vi "AquaLogic_Test_Stand.vi"() -> ()   [LabVIEW 2011]
panel:
  in  "Save Interval [s]":dbl=30.0 min=0.0
  in  "Save Enable":bool
  in  "STOP PROGRAM":bool
  in  "MAIN TAB":T1(tab)
  in  "?":T2={"ON-DEMAND Display"=[{"CMD_Display"="User Parameter : 20 Conductivity Thresholds", "Parameter Table"=[[">= Water Presence", ">= Low Salt", "<= Out of Salt [OFF]"], ["08.000", "10.000", "12.000"]], "SET"=FALSE, "GET"=FALSE}, {"CMD_Display"="User Parameter : 22 PCB Temp Threshold", "Parameter Table"=[[">= Max PCB Temp (°F)", "", ""], ["200.00", "", ""]], "SET"=FALSE, "GET"=FALSE}, {"CMD_Display"="User Parameter : 24 DayTank Setpoints", "Parameter Table"=[["<= Min / Empty Tank", ">= Fill Setpoint", ">= Tank Overfill"], ["00.500", "00.750", "01.250"]], "SET"=FALSE, "GET"=FALSE}, {"CMD_Display"="User Parameter : 25 Voltage Thresholds", "Parameter Table"=[["<= Min / Failure", ">= Low Salt", ">= Max / Failure"], ["00.000", "15.000", "20.000"]], "SET"=FALSE, "GET"=FALSE}, {"CMD_Display"="User Parameter : 26 Current Setpoint Limits", "Parameter Table"=[["Minimum Current (amps)", "Maximum Current (amps)", ""], ["00.000", "15.000", ""]], "SET"=FALSE, "GET"=FALSE}, {"CMD_Display"="User Parameter : 27 CURRCELL PWM Ramp", "Parameter Table"=[["Ramp Up Rate", "Ramp Down Rate", ""], ["00.250", "15.000", ""]], "SET"=FALSE, "GET"=FALSE}, {"CMD_Display"="User Parameter : 28 OUTPUT PWM Ramp", "Parameter Table"=[["Ramp Up Rate", "Ramp Down Rate", ""], ["00.500", "01.000", ""]], "SET"=FALSE, "GET"=FALSE}, {"CMD_Display"="User Parameter : 29 Cell Current SP / Status", "Parameter Table"=[["CURRCELL SP (amps)", "", ""], ["00.000", "", ""]], "SET"=FALSE, "GET"=FALSE}, {"CMD_Display"="User Parameter : 30 PWM Output 1 Setpoint", "Parameter Table"=[["Duty Cycle SP (%)", "", ""], ["0.00", "", ""]], "SET"=FALSE, "GET"=FALSE}, {"CMD_Display"="User Parameter : 31 PWM Output 2 Setpoint", "Parameter Table"=[["Duty Cycle SP (%)", "", ""], ["000.00", "", ""]], "SET"=FALSE, "GET"=FALSE}, {"CMD_Display"="User Parameter : 32 PWM Output 3 Setpoint", "Parameter Table"=[["Duty Cycle SP (%)", "", ""], ["000.00", "", ""]], "SET"=FALSE, "GET"=FALSE}], "CONTINUOUS Display"=[{"CMD_Display"="DU:33  Cell Status", "Param Output"=[["CELLDRIVE Duty (%)", "VOLTSCELL (volts)", "CURRCELL (amps)"], ["000.00", "00.000", "00.015"]]}, {"CMD_Display"="DU:34  PWM1 Status", "Param Output"=[["Duty Cycle (%)", "EMFOUT (volts)", "OVRCOUT (amps)"], ["000.00", "00.765", "00.000"]]}, {"CMD_Display"="DU:41  Temperature Measurements", "Param Output"=[["PCB Temperature (°F)", "Conductivity Temp (°F)", ""], ["069.91", "Conductivity Temp (°F)", ""]]}], "ERROR List"=[], "STATUS List"=[], "DIGITAL List"=[]}
  in  "Display B":T2={"ON-DEMAND Display"=[{"CMD_Display"="User Parameter : 20 Conductivity Thresholds", "Parameter Table"=[[">= Water Presence", ">= Low Salt", "<= Out of Salt [OFF]"], ["08.000", "10.000", "12.000"]], "SET"=FALSE, "GET"=FALSE}, {"CMD_Display"="User Parameter : 22 PCB Temp Threshold", "Parameter Table"=[[">= Max PCB Temp (°F)", "", ""], ["200.00", "", ""]], "SET"=FALSE, "GET"=FALSE}, {"CMD_Display"="User Parameter : 24 DayTank Setpoints", "Parameter Table"=[["<= Min / Empty Tank", ">= Fill Setpoint", ">= Tank Overfill"], ["00.500", "00.750", "01.250"]], "SET"=FALSE, "GET"=FALSE}, {"CMD_Display"="User Parameter : 25 Voltage Thresholds", "Parameter Table"=[["<= Min / Failure", ">= Low Salt", ">= Max / Failure"], ["00.000", "15.000", "20.000"]], "SET"=FALSE, "GET"=FALSE}, {"CMD_Display"="User Parameter : 26 Current Setpoint Limits", "Parameter Table"=[["Minimum Current (amps)", "Maximum Current (amps)", ""], ["00.000", "15.000", ""]], "SET"=FALSE, "GET"=FALSE}, {"CMD_Display"="User Parameter : 27 CURRCELL PWM Ramp", "Parameter Table"=[["Ramp Up Rate", "Ramp Down Rate", ""], ["00.250", "15.000", ""]], "SET"=FALSE, "GET"=FALSE}, {"CMD_Display"="User Parameter : 28 OUTPUT PWM Ramp", "Parameter Table"=[["Ramp Up Rate", "Ramp Down Rate", ""], ["00.500", "01.000", ""]], "SET"=FALSE, "GET"=FALSE}, {"CMD_Display"="User Parameter : 29 Cell Current SP / Status", "Parameter Table"=[["CURRCELL SP (amps)", "", ""], ["00.000", "", ""]], "SET"=FALSE, "GET"=FALSE}, {"CMD_Display"="User Parameter : 30 PWM Output 1 Setpoint", "Parameter Table"=[["Duty Cycle SP (%)", "", ""], ["0.00", "", ""]], "SET"=FALSE, "GET"=FALSE}, {"CMD_Display"="User Parameter : 31 PWM Output 2 Setpoint", "Parameter Table"=[["Duty Cycle SP (%)", "", ""], ["000.00", "", ""]], "SET"=FALSE, "GET"=FALSE}, {"CMD_Display"="User Parameter : 32 PWM Output 3 Setpoint", "Parameter Table"=[["Duty Cycle SP (%)", "", ""], ["000.00", "", ""]], "SET"=FALSE, "GET"=FALSE}], "CONTINUOUS Display"=[{"CMD_Display"="DU:33  Cell Status", "Param Output"=[["CELLDRIVE Duty (%)", "VOLTSCELL (volts)", "CURRCELL (amps)"], ["000.00", "00.000", "00.015"]]}, {"CMD_Display"="DU:34  PWM1 Status", "Param Output"=[["Duty Cycle (%)", "EMFOUT (volts)", "OVRCOUT (amps)"], ["000.00", "00.765", "00.000"]]}, {"CMD_Display"="DU:41  Temperature Measurements", "Param Output"=[["PCB Temperature (°F)", "Conductivity Temp (°F)", ""], ["069.91", "Conductivity Temp (°F)", ""]]}], "ERROR List"=[], "STATUS List"=[], "DIGITAL List"=[]}
  in  "Display C":T2={"ON-DEMAND Display"=[{"CMD_Display"="User Parameter : 20 Conductivity Thresholds", "Parameter Table"=[[">= Water Presence", ">= Low Salt", "<= Out of Salt [OFF]"], ["08.000", "10.000", "12.000"]], "SET"=FALSE, "GET"=FALSE}, {"CMD_Display"="User Parameter : 22 PCB Temp Threshold", "Parameter Table"=[[">= Max PCB Temp (°F)", "", ""], ["200.00", "", ""]], "SET"=FALSE, "GET"=FALSE}, {"CMD_Display"="User Parameter : 24 DayTank Setpoints", "Parameter Table"=[["<= Min / Empty Tank", ">= Fill Setpoint", ">= Tank Overfill"], ["00.500", "00.750", "01.250"]], "SET"=FALSE, "GET"=FALSE}, {"CMD_Display"="User Parameter : 25 Voltage Thresholds", "Parameter Table"=[["<= Min / Failure", ">= Low Salt", ">= Max / Failure"], ["00.000", "15.000", "20.000"]], "SET"=FALSE, "GET"=FALSE}, {"CMD_Display"="User Parameter : 26 Current Setpoint Limits", "Parameter Table"=[["Minimum Current (amps)", "Maximum Current (amps)", ""], ["00.000", "15.000", ""]], "SET"=FALSE, "GET"=FALSE}, {"CMD_Display"="User Parameter : 27 CURRCELL PWM Ramp", "Parameter Table"=[["Ramp Up Rate", "Ramp Down Rate", ""], ["00.250", "15.000", ""]], "SET"=FALSE, "GET"=FALSE}, {"CMD_Display"="User Parameter : 28 OUTPUT PWM Ramp", "Parameter Table"=[["Ramp Up Rate", "Ramp Down Rate", ""], ["00.500", "01.000", ""]], "SET"=FALSE, "GET"=FALSE}, {"CMD_Display"="User Parameter : 29 Cell Current SP / Status", "Parameter Table"=[["CURRCELL SP (amps)", "", ""], ["00.000", "", ""]], "SET"=FALSE, "GET"=FALSE}, {"CMD_Display"="User Parameter : 30 PWM Output 1 Setpoint", "Parameter Table"=[["Duty Cycle SP (%)", "", ""], ["0.00", "", ""]], "SET"=FALSE, "GET"=FALSE}, {"CMD_Display"="User Parameter : 31 PWM Output 2 Setpoint", "Parameter Table"=[["Duty Cycle SP (%)", "", ""], ["000.00", "", ""]], "SET"=FALSE, "GET"=FALSE}, {"CMD_Display"="User Parameter : 32 PWM Output 3 Setpoint", "Parameter Table"=[["Duty Cycle SP (%)", "", ""], ["000.00", "", ""]], "SET"=FALSE, "GET"=FALSE}], "CONTINUOUS Display"=[{"CMD_Display"="DU:33  Cell Status", "Param Output"=[["CELLDRIVE Duty (%)", "VOLTSCELL (volts)", "CURRCELL (amps)"], ["000.00", "00.000", "00.015"]]}, {"CMD_Display"="DU:34  PWM1 Status", "Param Output"=[["Duty Cycle (%)", "EMFOUT (volts)", "OVRCOUT (amps)"], ["000.00", "00.765", "00.000"]]}, {"CMD_Display"="DU:41  Temperature Measurements", "Param Output"=[["PCB Temperature (°F)", "Conductivity Temp (°F)", ""], ["069.91", "Conductivity Temp (°F)", ""]]}], "ERROR List"=[], "STATUS List"=[], "DIGITAL List"=[]}
  in  "Display D":T2={"ON-DEMAND Display"=[{"CMD_Display"="User Parameter : 20 Conductivity Thresholds", "Parameter Table"=[[">= Water Presence", ">= Low Salt", "<= Out of Salt [OFF]"], ["08.000", "10.000", "12.000"]], "SET"=FALSE, "GET"=FALSE}, {"CMD_Display"="User Parameter : 22 PCB Temp Threshold", "Parameter Table"=[[">= Max PCB Temp (°F)", "", ""], ["200.00", "", ""]], "SET"=FALSE, "GET"=FALSE}, {"CMD_Display"="User Parameter : 24 DayTank Setpoints", "Parameter Table"=[["<= Min / Empty Tank", ">= Fill Setpoint", ">= Tank Overfill"], ["00.500", "00.750", "01.250"]], "SET"=FALSE, "GET"=FALSE}, {"CMD_Display"="User Parameter : 25 Voltage Thresholds", "Parameter Table"=[["<= Min / Failure", ">= Low Salt", ">= Max / Failure"], ["00.000", "15.000", "20.000"]], "SET"=FALSE, "GET"=FALSE}, {"CMD_Display"="User Parameter : 26 Current Setpoint Limits", "Parameter Table"=[["Minimum Current (amps)", "Maximum Current (amps)", ""], ["00.000", "15.000", ""]], "SET"=FALSE, "GET"=FALSE}, {"CMD_Display"="User Parameter : 27 CURRCELL PWM Ramp", "Parameter Table"=[["Ramp Up Rate", "Ramp Down Rate", ""], ["00.250", "15.000", ""]], "SET"=FALSE, "GET"=FALSE}, {"CMD_Display"="User Parameter : 28 OUTPUT PWM Ramp", "Parameter Table"=[["Ramp Up Rate", "Ramp Down Rate", ""], ["00.500", "01.000", ""]], "SET"=FALSE, "GET"=FALSE}, {"CMD_Display"="User Parameter : 29 Cell Current SP / Status", "Parameter Table"=[["CURRCELL SP (amps)", "", ""], ["00.000", "", ""]], "SET"=FALSE, "GET"=FALSE}, {"CMD_Display"="User Parameter : 30 PWM Output 1 Setpoint", "Parameter Table"=[["Duty Cycle SP (%)", "", ""], ["0.00", "", ""]], "SET"=FALSE, "GET"=FALSE}, {"CMD_Display"="User Parameter : 31 PWM Output 2 Setpoint", "Parameter Table"=[["Duty Cycle SP (%)", "", ""], ["000.00", "", ""]], "SET"=FALSE, "GET"=FALSE}, {"CMD_Display"="User Parameter : 32 PWM Output 3 Setpoint", "Parameter Table"=[["Duty Cycle SP (%)", "", ""], ["000.00", "", ""]], "SET"=FALSE, "GET"=FALSE}], "CONTINUOUS Display"=[{"CMD_Display"="DU:33  Cell Status", "Param Output"=[["CELLDRIVE Duty (%)", "VOLTSCELL (volts)", "CURRCELL (amps)"], ["000.00", "00.000", "00.015"]]}, {"CMD_Display"="DU:34  PWM1 Status", "Param Output"=[["Duty Cycle (%)", "EMFOUT (volts)", "OVRCOUT (amps)"], ["000.00", "00.765", "00.000"]]}, {"CMD_Display"="DU:41  Temperature Measurements", "Param Output"=[["PCB Temperature (°F)", "Conductivity Temp (°F)", ""], ["069.91", "Conductivity Temp (°F)", ""]]}], "ERROR List"=[], "STATUS List"=[], "DIGITAL List"=[]}
  in  "CONTINUOUS Active Commands":i32[](array[numeric])=[33, 34, 38]
  in  "ON-DEMAND Config":bool
  in  "ON-DEMAND Active Commands":i32[](array[numeric])=[22, 25, 26, 27, 29, 30]
  in  "CONTINUOUS Config":bool
  in  "NEW CMD TABLE":i32[](listbox)=[-1]
  in  "ERROR Config":bool
  in  "STATUS Config":bool
  in  "DIGITAL Config":bool
  in  "ERROR Command":string="38"
  in  "STATUS Command":string="37"
  in  "DIGITAL Command":string="39"
  in  "Config Sub-Tab":T3(tab)=enum."General"
  out "ESP Error A":errorcluster={"status"=FALSE, "code"=1073676294, "source"="VISA Read in ESP-D Read-Write (SubVI).vi->CMD - On-Demand (SubVI).vi->AquaLogic_Test_Stand.vi"}
  out "ESP Output A":T4={"Write Command"="\u0001eb:DU:38:A600\u0004", "Read String"="", "Read Bytes"=0, "Bytes at Port"=0, "Response"="", "ACK"=FALSE, "EOT"=FALSE, "NAK"=FALSE, "Parameters"=[]}
  in  "ESP Config A":T5={"COM Port Input"="COM1", "Manual Command"={"Device Type"="", "Instance"="", "Command"="", "Sub-Command"="", "Parameters (Seperate by :)"=""}, "Device Type"="e", "Instance"="a", "Use Manual Command?"=FALSE, "Timeout [msec]"=1000, "Read/Write Wait [msec]"=25}
  out "ESP Error B":errorcluster={"status"=FALSE, "code"=1073676294, "source"="VISA Read in ESP-D Read-Write (SubVI).vi->CMD - On-Demand (SubVI).vi->AquaLogic_Test_Stand.vi"}
  out "ESP Output B":T4={"Write Command"="\u0001eb:DU:38:A600\u0004", "Read String"="", "Read Bytes"=0, "Bytes at Port"=0, "Response"="", "ACK"=FALSE, "EOT"=FALSE, "NAK"=FALSE, "Parameters"=[]}
  in  "ESP Config B":T5={"COM Port Input"="COM1", "Manual Command"={"Device Type"="", "Instance"="", "Command"="", "Sub-Command"="", "Parameters (Seperate by :)"=""}, "Device Type"="e", "Instance"="b", "Use Manual Command?"=FALSE, "Timeout [msec]"=1000, "Read/Write Wait [msec]"=25}
  out "ESP Error C":errorcluster={"status"=FALSE, "code"=1073676294, "source"="VISA Read in ESP-D Read-Write (SubVI).vi->CMD - On-Demand (SubVI).vi->AquaLogic_Test_Stand.vi"}
  out "ESP Output C":T4={"Write Command"="\u0001eb:DU:38:A600\u0004", "Read String"="", "Read Bytes"=0, "Bytes at Port"=0, "Response"="", "ACK"=FALSE, "EOT"=FALSE, "NAK"=FALSE, "Parameters"=[]}
  in  "ESP Config C":T5={"COM Port Input"="COM2", "Manual Command"={"Device Type"="", "Instance"="", "Command"="", "Sub-Command"="", "Parameters (Seperate by :)"=""}, "Device Type"="e", "Instance"="a", "Use Manual Command?"=FALSE, "Timeout [msec]"=1000, "Read/Write Wait [msec]"=25}
  out "ESP Error D":errorcluster={"status"=FALSE, "code"=1073676294, "source"="VISA Read in ESP-D Read-Write (SubVI).vi->CMD - On-Demand (SubVI).vi->AquaLogic_Test_Stand.vi"}
  out "ESP Output D":T4={"Write Command"="\u0001eb:DU:38:A600\u0004", "Read String"="", "Read Bytes"=0, "Bytes at Port"=0, "Response"="", "ACK"=FALSE, "EOT"=FALSE, "NAK"=FALSE, "Parameters"=[]}
  in  "ESP Config D":T5={"COM Port Input"="COM2", "Manual Command"={"Device Type"="", "Instance"="", "Command"="", "Sub-Command"="", "Parameters (Seperate by :)"=""}, "Device Type"="e", "Instance"="b", "Use Manual Command?"=FALSE, "Timeout [msec]"=1000, "Read/Write Wait [msec]"=25}
  in  "Folder Location":path
  out "Save Error":errorcluster
  in  "File Name":string
  in  "# of Active ESP Connections":i32=2
  in  "Loop Wait [ms]":u32=1
  out "Loop Time [ms]":u32=12368
  out "SYSTEM OK":bool
  # "AQUALOGIC \nLabVIEW Test Interface"
  # "Blake Otting - 2012"
  # "On-Demand ESP Commands (DU and SU)"
  # "Continuous-Read ESP Commands (DU)"
  # "On-Demand ESP Commands (DU and SU)"
  # "Continuous-Read ESP Commands (DU)"
  # "On-Demand ESP Commands (DU and SU)"
  # "Continuous-Read ESP Commands (DU)"
  # "On-Demand ESP Commands (DU and SU)"
  # "Continuous-Read ESP Commands (DU)"
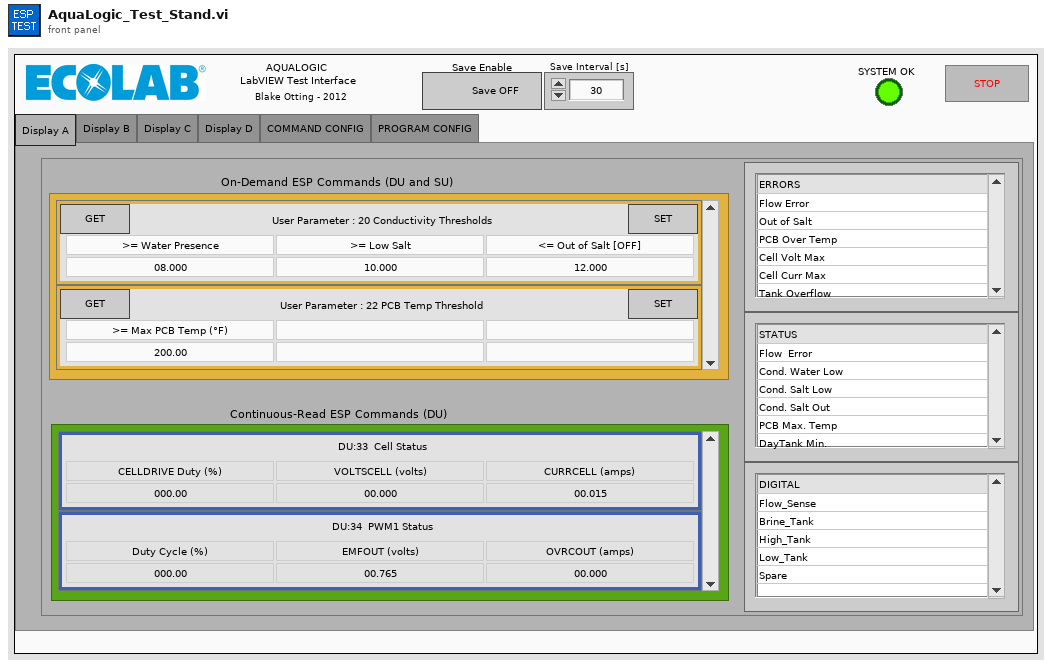
[diagram p1: front panel]
types:
  T1 = enum32{"Display A", "Display B", "Display C", "Display D", "COMMAND CONFIG", "PROGRAM CONFIG"}
  T2 = cluster{"ON-DEMAND Display":cluster{"CMD_Display":string, "Parameter Table":string[][], "SET":bool, "GET":bool}[], "CONTINUOUS Display":cluster{"CMD_Display":string, "Param Output":string[][]}[], "ERROR List":i32[], "STATUS List":i32[], "DIGITAL List":i32[]}
  T3 = enum32{"ESP A", "ESP B", "ESP C", "ESP D", "General", "Custom Display Parameters"}
  T4 = cluster{"Write Command":string, "Read String":string, "Read Bytes":u32, "Bytes at Port":u32, "Response":string, "ACK":bool, "EOT":bool, "NAK":bool, "Parameters":string[]}
  T5 = cluster{"COM Port Input":refnum<visa-resource-name>, "Manual Command":cluster{"Device Type":string, "Instance":string, "Command":string, "Sub-Command":string, "Parameters (Seperate by :)":string}, "Device Type":string, "Instance":string, "Use Manual Command?":bool, "Timeout [msec]":u32, "Read/Write Wait [msec]":u32}
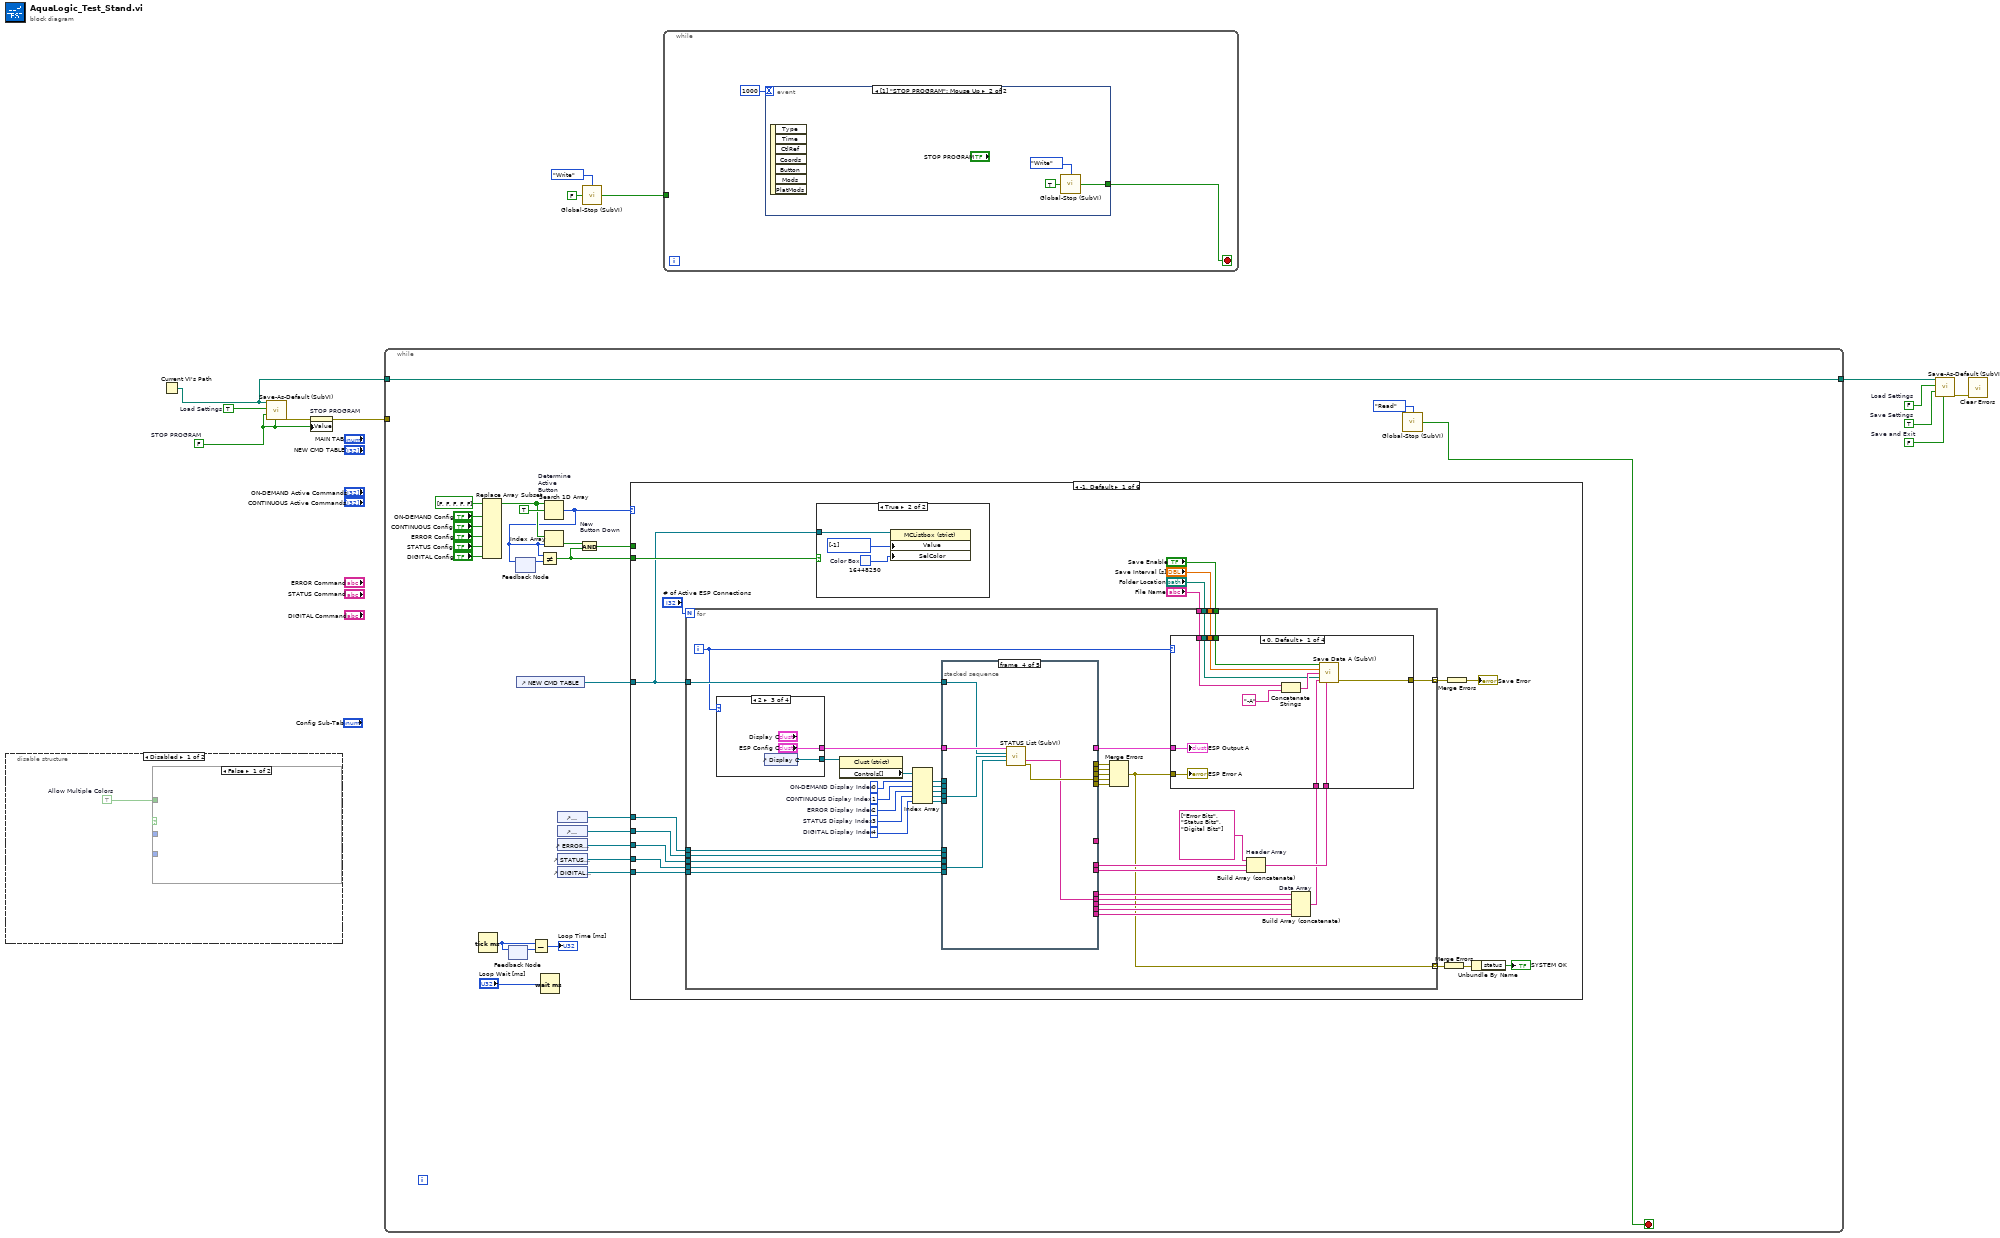
[diagram p0: block diagram]
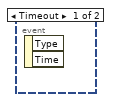
[diagram p2: hidden frame]
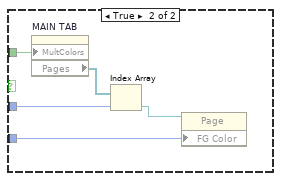
[diagram p3: hidden frame]
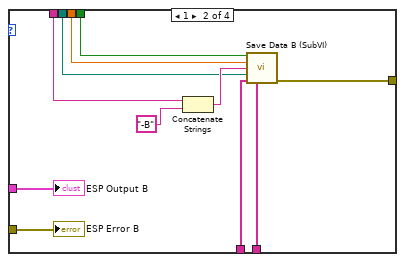
[diagram p5: hidden frame]
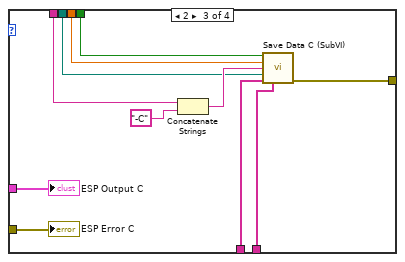
[diagram p6: hidden frame]
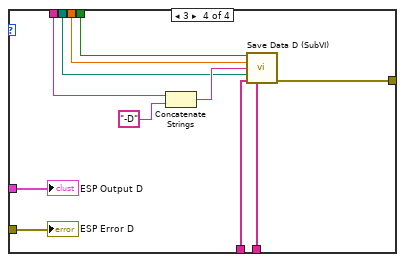
[diagram p7: hidden frame]
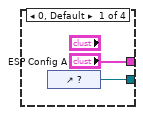
[diagram p8: hidden frame]
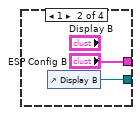
[diagram p9: hidden frame]
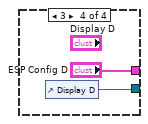
[diagram p10: hidden frame]
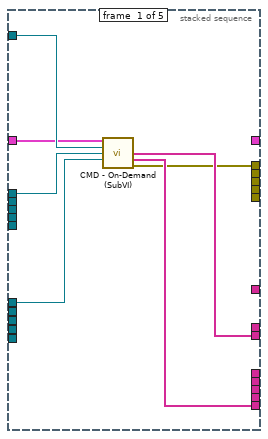
[diagram p11: hidden frame]
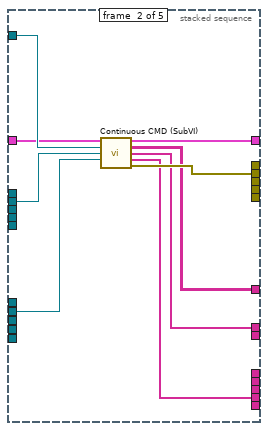
[diagram p12: hidden frame]
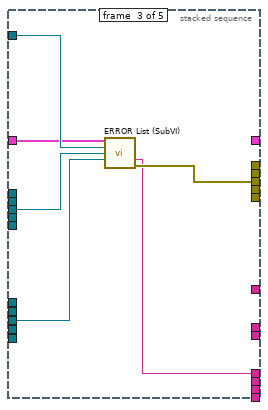
[diagram p13: hidden frame]
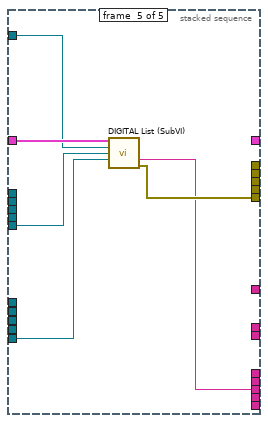
[diagram p14: hidden frame]
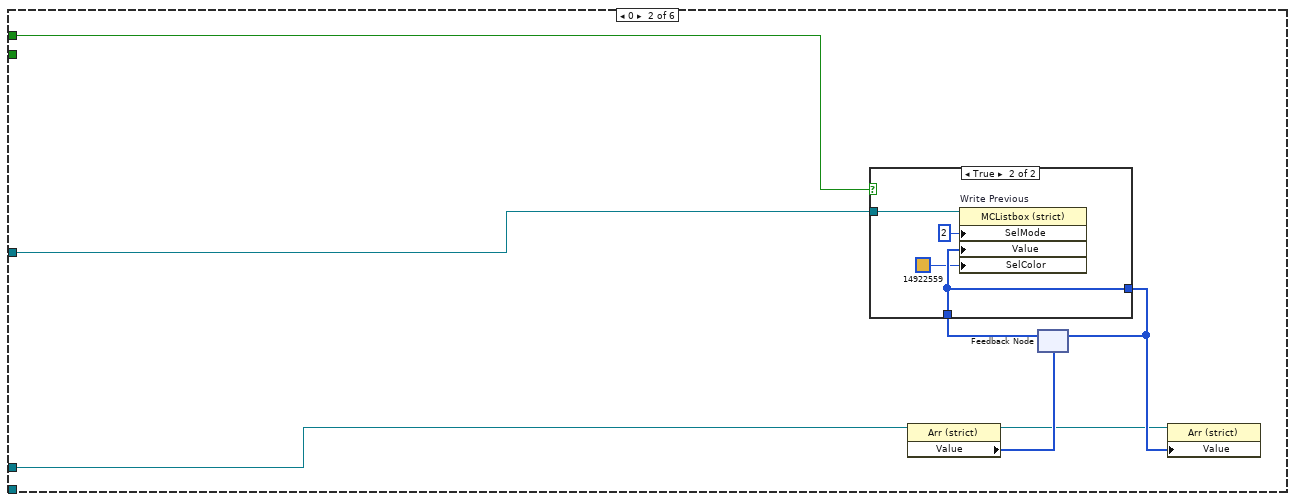
[diagram p16: hidden frame]
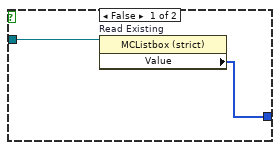
[diagram p17: hidden frame]
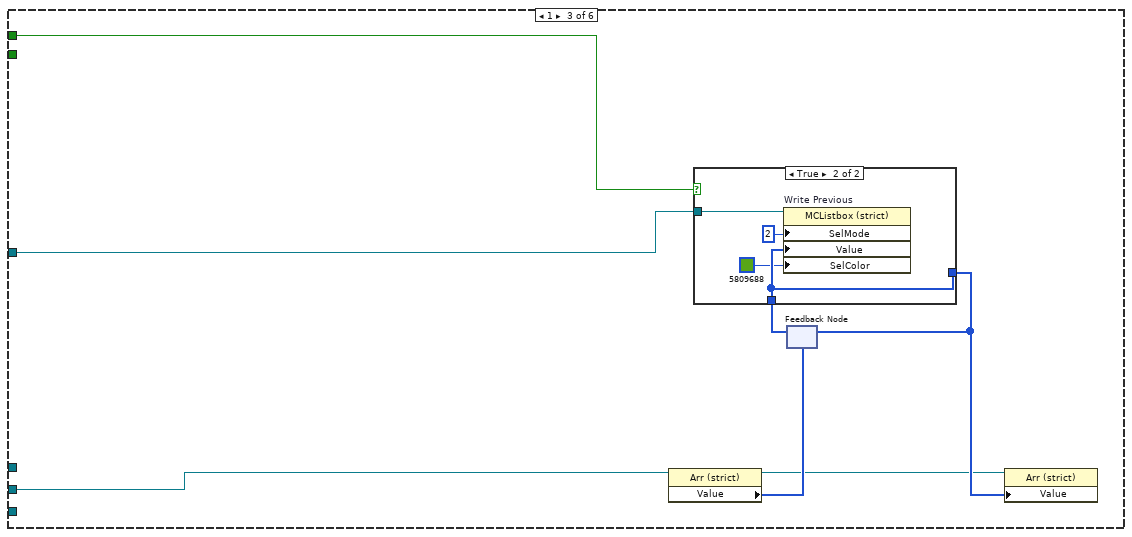
[diagram p18: hidden frame]
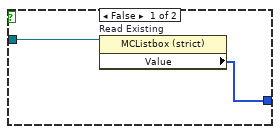
[diagram p19: hidden frame]
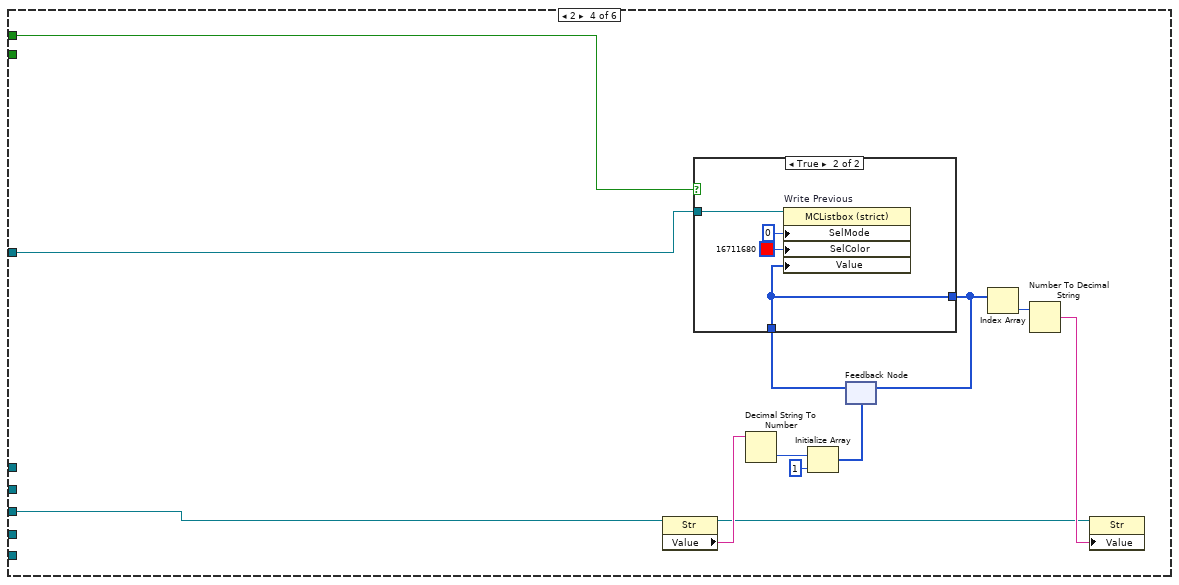
[diagram p20: hidden frame]
diagram:
  w5 = FALSE  # Save and Exit
  w6 = TRUE  # Save Settings
  w7 = FALSE  # Load Settings
  w12 = TRUE  # Load Settings
  w10 = FALSE  # STOP PROGRAM
  n1 = disable-structure shown="Disabled" {
    frame Disabled {
      w14 = TRUE  # Allow Multiple Colors
      n2 = case shown="False" {
        selector: _ -> [_ _]
        tunnel: w14 -> [_ w21]
        tunnel: [_ w19] -> w15
        tunnel: [_ w17] -> w16
        frame False {
        }
        frame True {
          n3 = property on="MAIN TAB" class="TabCtl (strict)"("MultColors"=w21) -> ("Pages"=w20:refnum<vi>[])  [unwired: 2 in, 2 out]
          n4 = Index Array(array=w20, index=w19) -> (element=w18:refnum<vi>)
          n5 = property class="Page"(reference=w18, "FG Color"=w17) -> ()  [unwired: 1 in, 2 out]
        }
      }
    }
    frame Enabled {
    }
  }
  n6 = Current VI's Path() -> (path=w9:path)
  n7 = call "Save-As-Default (SubVI).vi"("Current VI's Path"=w9, "Load Settings"=w12, "Save Settings"=w10, "Save and Exit"=w10) -> ("Save as Default Error"=w11:errorcluster)  [unwired: 15 in]
  n8 = property on="STOP PROGRAM" class="Bool (strict)"(error in=w11, "Value"=w10) -> (error out=w13:errorcluster)  [unwired: 1 in, 1 out]
  n9 = while {
    tunnel: w13 -> [_]
    tunnel: w9 -> [w25]
    tunnel: [w25] -> w8
    stop <- w22 stop-if-true
    n10 = Tick Count (ms)() -> (millisecond timer value=w28:u32)
    n11 = Replace Array Subset(array=bool[] [FALSE, FALSE, FALSE, FALSE, FALSE], new element #1="ON-DEMAND Config", new element #2="CONTINUOUS Config", new element #3="ERROR Config", new element #4="STATUS Config", new element #5="DIGITAL Config") -> (w39:bool[])  [unwired: 5 in]
    n12 = feedback-in #1(w28) -> ()
    n13 = feedback #1() -> (w27:u32)  [unwired: 1 in]
    n14 = feedback #2() -> (w40:i32)  [unwired: 1 in]
    n15 = control-ref of="NEW CMD TABLE"() -> (w29:refnum<vi>)
    n16 = Subtract(x=w28, y=w27) -> (x-y=→"Loop Time [ms]":u32)
    n17 = Wait (ms)(milliseconds to wait="Loop Wait [ms]") -> ()  [unwired: 1 out]
    n18 = Search 1D Array "Determine\nActive\nButton"(1D array=w39, element=TRUE) -> (index of element=w30:i32)  [unwired: 1 in]
    n19 = feedback-in #2(w30) -> ()
    n20 = Not Equal?(x=w30, y=w40) -> (x != y?=w36:bool)
    n21 = Index Array(array=w39, index=w30) -> (element=w37:bool)
    n22 = control-ref of="ON-DEMAND Active Commands"() -> (w35:refnum<vi>)
    n23 = control-ref of="CONTINUOUS Active Commands"() -> (w34:refnum<vi>)
    n24 = control-ref of="ERROR Command"() -> (w33:refnum<vi>)
    n25 = control-ref of="STATUS Command"() -> (w32:refnum<vi>)
    n26 = control-ref of="DIGITAL Command"() -> (w31:refnum<vi>)
    n27 = And "New\nButton Down"(x=w37, y=w36) -> (x .and. y?=w38:bool)
    n28 = case shown="-1, Default" w30 {
      tunnel: w38 -> [_ w202 w214 w232 w250 w268]
      tunnel: w36 -> [w64 _ _ _ _ _]
      tunnel: w29 -> [w58 w199 w212 w228 w246 w264]
      tunnel: w35 -> [w63 w198 _ _ _ _]
      tunnel: w34 -> [w62 _ w211 _ _ _]
      tunnel: w33 -> [w61 _ _ w226 _ _]
      tunnel: w32 -> [w60 _ _ _ w242 _]
      tunnel: w31 -> [w59 _ _ _ _ w260]
      frame -1, Default {
        n29 = for {
          N: "# of Active ESP Connections" -> [_]
          tunnel: w63 -> [w106]
          tunnel: w62 -> [w105]
          tunnel: w61 -> [w104]
          tunnel: w60 -> [w103]
          tunnel: w59 -> [w102]
          tunnel: w58 -> [w101]
          tunnel: "File Name" -> [w76]
          tunnel: "Folder Location" -> [w75]
          tunnel: "Save Interval [s]" -> [w74]
          tunnel: "Save Enable" -> [w73]
          tunnel: [w72] -> w51 mode=indexing
          tunnel: [w65] -> w49 mode=indexing
          i -> [w71]
          w83 = 4  # DIGITAL Display Index
          w84 = 3  # STATUS Display Index
          w85 = 2  # ERROR Display Index
          w86 = 1  # CONTINUOUS Display Index
          w87 = 0  # ON-DEMAND Display Index
          n30 = case shown="2" w71 {
            tunnel: [w152 w153 w155 w157] -> w70
            tunnel: ["ESP Config A" "ESP Config B" "ESP Config C" "ESP Config D"] -> w69
            frame 0, Default {
              n31 = control-ref of="?"() -> (w152:refnum<vi>)
            }
            frame 1 {
              n32 = control-ref of="Display B"() -> (w153:refnum<vi>)
            }
            frame 2 {
              n33 = control-ref of="Display C"() -> (w155:refnum<vi>)
            }
            frame 3 {
              n34 = control-ref of="Display D"() -> (w157:refnum<vi>)
            }
          }
          n35 = property class="Clust (strict)"(reference=w70) -> ("Controls[]"=w77:refnum<vi>[])  [unwired: 1 in, 2 out]
          n36 = Index Array(array=w77, index #1=w87, index #2=w86, index #3=w85, index #4=w84, index #5=w83) -> (element #1=w82:refnum<vi>, element #2=w81:refnum<vi>, element #3=w80:refnum<vi>, element #4=w79:refnum<vi>, element #5=w78:refnum<vi>)
          n37 = stacked-sequence {
            tunnel: w101 -> [w165 w174 w179 w184 w190]
            tunnel: w69 -> [w164 w173 w178 w185 w191]
            tunnel: w106 -> [w163 _ _ _ _]
            tunnel: [w159 _ _ _ _] -> w100
            tunnel: [_ w172 _ _ _] -> w99
            tunnel: [_ _ w180 _ _] -> w98
            tunnel: [_ _ _ w186 _] -> w97
            tunnel: [_ _ _ _ w192] -> w96
            tunnel: w105 -> [_ w171 _ _ _]
            tunnel: w104 -> [_ _ w177 _ _]
            tunnel: w103 -> [_ _ _ w183 _]
            tunnel: w102 -> [_ _ _ _ w189]
            tunnel: [_ w169 _ _ _] -> _
            tunnel: [_ w170 _ _ _] -> w95
            tunnel: [w162 _ _ _ _] -> w93
            tunnel: [_ w168 _ _ _] -> w94
            tunnel: [_ w167 _ _ _] -> w89
            tunnel: [_ _ w176 _ _] -> w92
            tunnel: [w161 _ _ _ _] -> w88
            tunnel: [_ _ _ w182 _] -> w91
            tunnel: [_ _ _ _ w188] -> w90
            tunnel: w82 -> [w160 _ _ _ _]
            tunnel: w81 -> [_ w166 _ _ _]
            tunnel: w80 -> [_ _ w175 _ _]
            tunnel: w79 -> [_ _ _ w181 _]
            tunnel: w78 -> [_ _ _ _ w187]
            frame #0 {
              n38 = call "CMD - On-Demand (SubVI).vi"("ESP Config"=w164, "Command Table Ref"=w165, "ON-DEMAND Ref"=w160, "ON-DEMAND Active Commands Ref"=w163) -> ("On-Demand Header"=w162:string[], "On-Demand Data"=w161:string[], "ON Demand"=w159:errorcluster)  [unwired: 8 in, 1 out]
            }
            frame #1 {
              n39 = call "Continuous CMD (SubVI).vi"("ESP Config"=w173, "Command Table Ref"=w174, "CONTINUOUS Display Ref"=w166, "CONTINUOUS Active Commands"=w171) -> ("ESP Values"=w170:T4, "Parameters"=w169:string[][], "Continuous Header"=w168:string[], "Continuous Data"=w167:string[], "CONTINUOUS"=w172:errorcluster)  [unwired: 7 in]
            }
            frame #2 {
              n40 = call "ERROR List (SubVI).vi"("ESP Config"=w178, "Command Table Ref IN"=w179, "ERROR Display Ref"=w175, "ERROR Command Ref"=w177) -> ("Error Data"=w176:string, "ERROR List"=w180:errorcluster)  [unwired: 10 in]
            }
            frame #3 {
              n41 = call "STATUS List (SubVI).vi"("ESP Config"=w185, "Command Table Ref"=w184, "STATUS Display Ref"=w181, "STATUS Command Ref"=w183) -> ("Status Data"=w182:string, "STATUS List"=w186:errorcluster)  [unwired: 10 in]
            }
            frame #4 {
              n42 = call "DIGITAL List (SubVI).vi"("ESP Config"=w191, "Command Table Ref"=w190, "DIGITAL Display Ref"=w187, "DIGITAL Command Ref"=w189) -> ("Digital Data"=w188:string, "DIGITAL List"=w192:errorcluster)  [unwired: 10 in]
            }
          }
          n43 = Merge Errors(w100, w99, w98, w97, w96) -> (w72:errorcluster)
          n44 = Build Array (concatenate) "Header Array"(string[] ["Error Bits", "Status Bits", "Digital Bits"], w94, w93) -> (w67:string[])
          n45 = Build Array (concatenate) "Data Array"(w92, w91, w90, w89, w88) -> (w66:string[])
          n46 = case shown="0, Default" w71 {
            tunnel: w95 -> [w117 w128 w139 w150]
            tunnel: w72 -> [w116 w127 w138 w149]
            tunnel: w76 -> [w114 w125 w131 w140]
            tunnel: w75 -> [w112 w118 w129 w141]
            tunnel: w74 -> [w111 w119 w136 w144]
            tunnel: w73 -> [w110 w121 w137 w145]
            tunnel: w67 -> [w109 w122 w133 w147]
            tunnel: w66 -> [w108 w123 w135 w148]
            tunnel: [w107 w120 w134 w146] -> w65
            frame 0, Default {
              n47 = Concatenate Strings(w114, "-A") -> (w113:string)
              n48 = call "Save Data A (SubVI).vi"("Save Enable"=w110, "Save Interval [s]"=w111, "File Name"=w113, "Folder Location"=w112, "Data Array (Row)"=w108, "Column Header Array"=w109) -> ("Save Error"=w107:errorcluster)  [unwired: 7 in, 2 out]
              "ESP Output A" <- w117
              "ESP Error A" <- w116
            }
            frame 1 {
              n49 = Concatenate Strings(w125, "-B") -> (w124:string)
              n50 = call "Save Data B (SubVI).vi"("Save Enable"=w121, "Save Interval [s]"=w119, "File Name"=w124, "Folder Location"=w118, "Data Array (Row)"=w123, "Column Header Array"=w122) -> ("Save Error"=w120:errorcluster)  [unwired: 7 in, 2 out]
              "ESP Error B" <- w127
              "ESP Output B" <- w128
            }
            frame 2 {
              n51 = Concatenate Strings(w131, "-C") -> (w130:string)
              n52 = call "Save Data C (SubVI).vi"("Save Enable"=w137, "Save Interval [s]"=w136, "File Name"=w130, "Folder Location"=w129, "Data Array (Row)"=w135, "Column Header Array"=w133) -> ("Save Error"=w134:errorcluster)  [unwired: 7 in, 2 out]
              "ESP Error C" <- w138
              "ESP Output C" <- w139
            }
            frame 3 {
              n53 = Concatenate Strings(w140, "-D") -> (w142:string)
              n54 = call "Save Data D (SubVI).vi"("Save Enable"=w145, "Save Interval [s]"=w144, "File Name"=w142, "Folder Location"=w141, "Data Array (Row)"=w148, "Column Header Array"=w147) -> ("Save Error"=w146:errorcluster)  [unwired: 7 in, 2 out]
              "ESP Output D" <- w150
              "ESP Error D" <- w149
            }
          }
        }
        n55 = case shown="True" w64 {
          tunnel: w58 -> [_ w195]
          frame False {
          }
          frame True {
            w193 = u32 16448250  # Color Box
            n56 = property class="MCListbox (strict)"(reference=w195, "Value"=i32[] [-1], "SelColor"=w193) -> ()  [unwired: 1 in, 2 out]
          }
        }
        n57 = Merge Errors(w51) -> (w50:errorcluster)
        n58 = Merge Errors(w49) -> (→"Save Error":errorcluster)
        n59 = Unbundle By Name(w50) -> ("status"=→"SYSTEM OK":bool)
      }
      frame 0 {
        n60 = property class="Arr (strict)"(reference=w198) -> (reference out=w196:refnum<vi>, "Value"=w197:i32[])  [unwired: 1 in, 1 out]
        n61 = feedback #3(w197) -> (w201:i32[])
        n62 = case shown="True" w202 {
          tunnel: w199 -> [w204 w208]
          tunnel: [w203 w207] -> w200
          tunnel: w201 -> [_ w207]
          frame False {
            n63 = property on="Read Existing" class="MCListbox (strict)"(reference=w204) -> ("Value"=w203:i32[])  [unwired: 1 in, 2 out]
          }
          frame True {
            n64 = property on="Write Previous" class="MCListbox (strict)"(reference=w208, "SelMode"=2, "Value"=w207, "SelColor"=u32 14922559) -> ()  [unwired: 1 in, 2 out]
          }
        }
        n65 = feedback-in #3(w200) -> ()
        n66 = property class="Arr (strict)"(reference=w196, "Value"=w200) -> ()  [unwired: 1 in, 2 out]
      }
      frame 1 {
        n67 = property class="Arr (strict)"(reference=w211) -> (reference out=w209:refnum<vi>, "Value"=w210:i32[])  [unwired: 1 in, 1 out]
        n68 = feedback #4(w210) -> (w215:i32[])
        n69 = case shown="True" w214 {
          tunnel: w212 -> [w217 w221]
          tunnel: [w216 w220] -> w213
          tunnel: w215 -> [_ w220]
          frame False {
            n70 = property on="Read Existing" class="MCListbox (strict)"(reference=w217) -> ("Value"=w216:i32[])  [unwired: 1 in, 2 out]
          }
          frame True {
            n71 = property on="Write Previous" class="MCListbox (strict)"(reference=w221, "SelMode"=2, "Value"=w220, "SelColor"=u32 5809688) -> ()  [unwired: 1 in, 2 out]
          }
        }
        n72 = feedback-in #4(w213) -> ()
        n73 = property class="Arr (strict)"(reference=w209, "Value"=w213) -> ()  [unwired: 1 in, 2 out]
      }
      frame 2 {
        n74 = property class="Str"(reference=w226) -> (reference out=w222:refnum<vi>, "Value"=w227:string)  [unwired: 1 in, 1 out]
        n75 = Decimal String To Number(string=w227) -> (number=w224:i32)  [unwired: 2 in, 1 out]
        n76 = Initialize Array(w224, 1) -> (w223:i32[])
        n77 = feedback #5(w223) -> (w233:i32[])
        n78 = case shown="True" w232 {
          tunnel: w228 -> [w235 w239]
          tunnel: [w234 w236] -> w231
          tunnel: w233 -> [_ w236]
          frame False {
            n79 = property on="Read Existing" class="MCListbox (strict)"(reference=w235) -> ("Value"=w234:i32[])  [unwired: 1 in, 2 out]
          }
          frame True {
            n80 = property on="Write Previous" class="MCListbox (strict)"(reference=w239, "SelMode"=0, "SelColor"=u32 16711680, "Value"=w236) -> ()  [unwired: 1 in, 2 out]
          }
        }
        n81 = feedback-in #5(w231) -> ()
        n82 = Index Array(array=w231) -> (element=w230:i32)  [unwired: 1 in]
        n83 = Number To Decimal String(number=w230) -> (decimal integer string=w229:string)  [unwired: 1 in]
        n84 = property class="Str"(reference=w222, "Value"=w229) -> ()  [unwired: 1 in, 2 out]
      }
      frame 3 {
        n85 = property class="Str"(reference=w242) -> (reference out=w241:refnum<vi>, "Value"=w245:string)  [unwired: 1 in, 1 out]
        n86 = Decimal String To Number(string=w245) -> (number=w243:i32)  [unwired: 2 in, 1 out]
        n87 = Initialize Array(w243, 1) -> (w240:i32[])
        n88 = feedback #6(w240) -> (w251:i32[])
        n89 = case shown="True" w250 {
          tunnel: w246 -> [w253 w257]
          tunnel: [w252 w254] -> w249
          tunnel: w251 -> [_ w254]
          frame False {
            n90 = property on="Read Existing" class="MCListbox (strict)"(reference=w253) -> ("Value"=w252:i32[])  [unwired: 1 in, 2 out]
          }
          frame True {
            n91 = property on="Write Previous" class="MCListbox (strict)"(reference=w257, "SelMode"=0, "SelColor"=u32 39372, "Value"=w254) -> ()  [unwired: 1 in, 2 out]
          }
        }
        n92 = feedback-in #6(w249) -> ()
        n93 = Index Array(array=w249) -> (element=w248:i32)  [unwired: 1 in]
        n94 = Number To Decimal String(number=w248) -> (decimal integer string=w247:string)  [unwired: 1 in]
        n95 = property class="Str"(reference=w241, "Value"=w247) -> ()  [unwired: 1 in, 2 out]
      }
      frame 4 {
        n96 = property class="Str"(reference=w260) -> (reference out=w259:refnum<vi>, "Value"=w263:string)  [unwired: 1 in, 1 out]
        n97 = Decimal String To Number(string=w263) -> (number=w261:i32)  [unwired: 2 in, 1 out]
        n98 = Initialize Array(w261, 1) -> (w258:i32[])
        n99 = feedback #7(w258) -> (w269:i32[])
        n100 = case shown="False" w268 {
          tunnel: w264 -> [w273 w279]
          tunnel: [w272 w274] -> w267
          tunnel: w269 -> [_ w274]
          tunnel: [w270 w278] -> _
          tunnel: [w271 w277] -> _
          frame False {
            n101 = property on="Read Existing" class="MCListbox (strict)"(reference=w273) -> (reference out=w270:refnum<vi>, error out=w271:errorcluster, "Value"=w272:i32[])  [unwired: 1 in]
          }
          frame True {
            n102 = property on="Write Previous" class="MCListbox (strict)"(reference=w279, "SelMode"=0, "SelColor"=u32 8421631, "Value"=w274) -> (reference out=w278:refnum<vi>, error out=w277:errorcluster)  [unwired: 1 in]
          }
        }
        n103 = feedback-in #7(w267) -> ()
        n104 = Index Array(array=w267) -> (element=w266:i32)  [unwired: 1 in]
        n105 = Number To Decimal String(number=w266) -> (decimal integer string=w265:string)  [unwired: 1 in]
        n106 = property class="Str"(reference=w259, "Value"=w265) -> ()  [unwired: 1 in, 2 out]
      }
    }
    n107 = call "Global-Stop (SubVI).vi"("Mode (Read)"=enum16{"Read", "Write"}."Read") -> ("OUT"=w22:bool)  [unwired: 3 in]
  }
  n108 = call "Global-Stop (SubVI).vi"("Mode (Read)"=enum16{"Read", "Write"}."Write", "IN"=FALSE) -> ("OUT"=w1:bool)  [unwired: 2 in]
  n109 = while {
    tunnel: w1 -> [_]
    stop <- w281 stop-if-true
    n110 = event shown="[1] \"STOP PROGRAM\": Mouse Up" {
      selector: _ -> [_ _]
      dyn-events: _ -> [_ _]
      timeout: 1000 -> [_ _]
      tunnel: [_ w284] -> w281
      event Timeout {
        n111 = event-data() -> ()  [unwired: 1 in, 2 out]
      }
      event "STOP PROGRAM": Mouse Up {
        n112 = event-data() -> ()  [unwired: 1 in, 7 out]
        n113 = call "Global-Stop (SubVI).vi"("Mode (Read)"=enum16{"Read", "Write"}."Write", "IN"=TRUE) -> ("OUT"=w284:bool)  [unwired: 2 in]
      }
    }
  }
  n114 = call "Save-As-Default (SubVI).vi"("Current VI's Path"=w8, "Load Settings"=w7, "Save Settings"=w6, "Save and Exit"=w5) -> ("Save as Default Error"=w4:errorcluster)  [unwired: 15 in]
  n115 = call <vilib>:"Clear Errors.vi"("error in (no error)"=w4) -> ()  [unwired: 6 in, 1 out]
